vi "Log.vi"(10 "Log Packet":T1, 11 "ConsoleSink in":refnum<class "ConsoleSink.lvclass">) -> (0 "error out":errorcluster, 3 "ConsoleSink out":refnum<class "ConsoleSink.lvclass">)   [LabVIEW 2019, in "ConsoleView.lvlib" / "ConsoleSink.lvclass"]
uses:
  <vilib>/gpm_packages/@cs/event-logger/Source/ConsoleView/Sink/ConsoleSink.lvclass
  <vilib>/gpm_packages/@cs/event-logger/Source/Composed Log/Types/Log Packet.ctl
  <vilib>/gpm_packages/@cs/event-logger/Source/Composed Log/Types/Log Level.ctl
  <vilib>/gpm_packages/@cs/event-logger/Source/ConsoleView/Sink/ConsoleSink.lvclass/ConsoleSink.ctl
  <vilib>/gpm_packages/@cs/event-logger/Source/Composed Log/Types/MessageCluster.ctl
  <vilib>/gpm_packages/@cs/event-logger/Source/Composed Log/Composed Log.lvlib
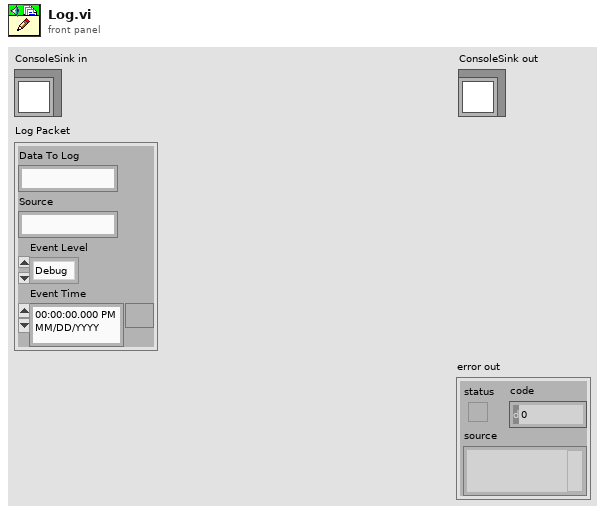
[diagram p1: front panel]
types:
  T1 = typedef "Composed Log.lvlib/Log Packet.ctl" = cluster{"Data To Log":string, "Source":string, "Event Level":T2, "Event Time":timestamp}
  T2 = typedef "Composed Log.lvlib/Log Level.ctl" = enum16{"Debug", "Info", "Warning", "Error", "Critical"}
  T3 = typedef "Composed Log.lvlib/MessageCluster.ctl" = cluster{"Message":string, "Data":variant}
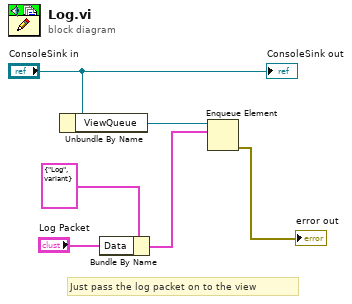
[diagram p0: block diagram]
diagram:
  # "Just pass the log packet on to the view"
  n1 = Unbundle By Name("ConsoleSink in") -> ("ViewQueue"=w5:refnum<queue>)
  n2 = Bundle By Name(cluster=T3 {"Message"="Log", "Data"=variant} ("element"), "Data"="Log Packet") -> (w3:T3)
  n3 = Enqueue Element(queue=w5, element=w3) -> (error out=→"error out":errorcluster)  [unwired: 2 in, 2 out]
  "ConsoleSink out" <- "ConsoleSink in"
